vi "set_up_graph_control_properties.vi"(9 "Graph Properties":T2, 10 "viewing volume":dbl[](array[numeric]), 11 "3D Picture Control Reference":refnum<vi>) -> ()   [LabVIEW 2020, in "3DPC_SurfacePlot.xctl"]
uses:
  <vilib>/Native 3D Graph/xcontrol/3DPC_SurfacePlot.xctl
  <vilib>/Native 3D Graph/typedefs/prop_graph.ctl
  <vilib>/picture/3D Picture Control/NI_3D Picture Control.lvlib
panel:
  in  "View Direction":T1(ring)
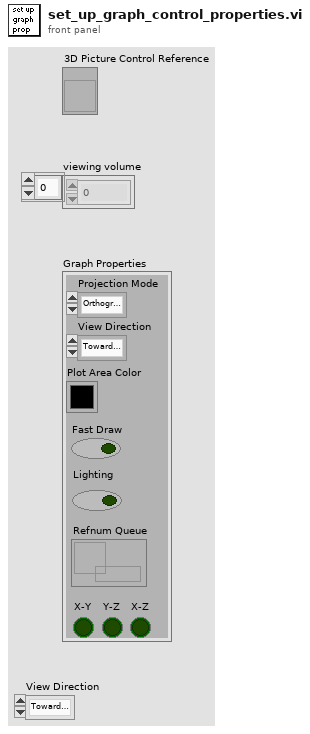
[diagram p1: front panel]
types:
  T1 = enum32{"Towards X-Y Plane", "Towards Y-Z Plane", "Towards X-Z Plane", "User Define"}
  T2 = typedef "3DPC_SurfacePlot.xctl/prop_graph.ctl" = cluster{"Projection Mode":enum16{"Orthographic", "Perspective"}, "View Direction":enum32{"Towards X-Y Plane", "Towards Y-Z Plane", "Towards X-Z Plane", "User Define"}, "Plot Area Color":u32, "Fast Draw":bool, "X-Y":bool, "Y-Z":bool, "X-Z":bool, "Lighting":bool, "Refnum Queue":refnum<queue>}
  T3 = enum16{"None", "Spherical", "Flying", "Oriented"}
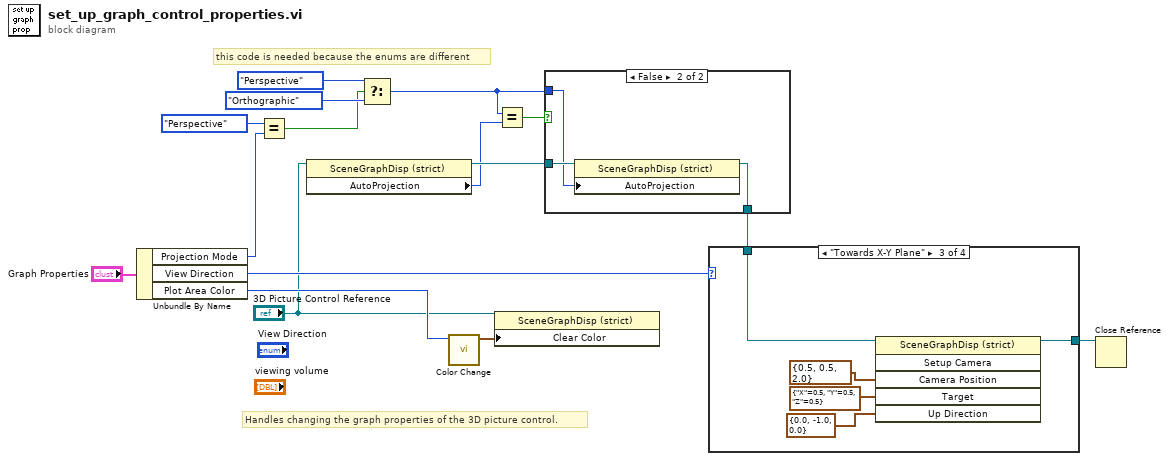
[diagram p0: block diagram]
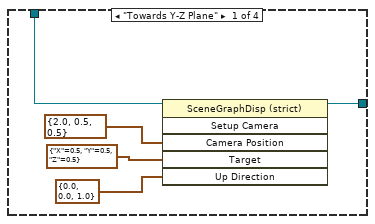
[diagram p2: hidden frame]
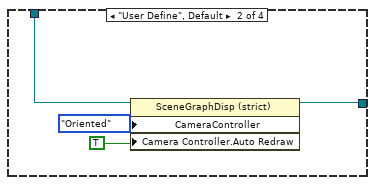
[diagram p3: hidden frame]
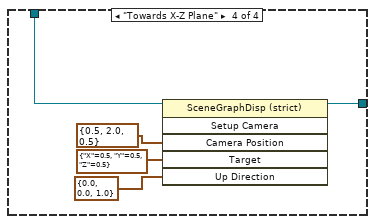
[diagram p4: hidden frame]
diagram:
  # "this code is needed because the enums are different"
  # "Handles changing the graph properties of the 3D picture control."
  n1 = Unbundle By Name("Graph Properties") -> ("Projection Mode"=w6:enum16{"Orthographic", "Perspective"}, "View Direction"=w15:T1, "Plot Area Color"=w14:u32)
  n2 = Equal?(x=enum16{"Orthographic", "Perspective"}."Perspective", y=w6) -> (x = y?=w4:bool)
  n3 = property class="SceneGraphDisp (strict)"(reference="3D Picture Control Reference") -> (reference out=w10:refnum<vi>, "AutoProjection"=w3:enum16{"None", "Perspective", "Orthographic"})  [unwired: 1 in, 1 out]
  n4 = Select(t=enum16{"None", "Perspective", "Orthographic"}."Perspective" ("Automatic Projection Mode"), s=w4, f=enum16{"None", "Perspective", "Orthographic"}."Orthographic" ("Automatic Projection Mode")) -> (s? t:f=w1:enum16{"None", "Perspective", "Orthographic"})
  n5 = call <vilib>:"Color Change.vi"("Color"=w14) -> ("RGBA"=w13:cluster{"R":sgl, "G":sgl, "B":sgl, "A":sgl})  [unwired: 1 in, 9 out]
  n6 = property on="Property Node" class="SceneGraphDisp (strict)"(reference="3D Picture Control Reference", "Clear Color"=w13) -> ()  [unwired: 1 in, 2 out]
  n7 = Equal?(x=w1, y=w3) -> (x = y?=w12:bool)
  n8 = case shown="False" w12 {
    tunnel: [w17 w18] -> w9
    tunnel: w10 -> [w17 w20]
    tunnel: w1 -> [_ w19]
    frame True {
    }
    frame False {
      n9 = property class="SceneGraphDisp (strict)"(reference=w20, "AutoProjection"=w19) -> (reference out=w18:refnum<vi>)  [unwired: 1 in, 1 out]
    }
  }
  n10 = case shown="\"Towards X-Y Plane\"" w15 {
    tunnel: [w22 w27 w30 w35] -> w2
    tunnel: w9 -> [w21 w28 w31 w36]
    frame "Towards Y-Z Plane" {
      n11 = invoke class="SceneGraphDisp (strict)" method="Setup Camera"(reference=w21, "Camera Position"=cluster{"X":sgl, "Y":sgl, "Z":sgl} {"X"=2.0, "Y"=0.5, "Z"=0.5}, "Target"=cluster{"X":sgl, "Y":sgl, "Z":sgl} {"X"=0.5, "Y"=0.5, "Z"=0.5} ("Camera Position"), "Up Direction"=cluster{"X":sgl, "Y":sgl, "Z":sgl} {"X"=0.0, "Y"=0.0, "Z"=1.0} ("Camera Position")) -> (reference out=w22:refnum<vi>)  [unwired: 2 in, 5 out]
    }
    frame "User Define", Default {
      n12 = property class="SceneGraphDisp (strict)"(reference=w28, "CameraController"=T3."Oriented" ("Camera Controller:Type"), "Camera Controller.Auto Redraw"=TRUE ("Camera Controller:Auto Redraw")) -> (reference out=w27:refnum<vi>)  [unwired: 1 in, 1 out]
    }
    frame "Towards X-Y Plane" {
      n13 = invoke class="SceneGraphDisp (strict)" method="Setup Camera"(reference=w31, "Camera Position"=cluster{"X":sgl, "Y":sgl, "Z":sgl} {"X"=0.5, "Y"=0.5, "Z"=2.0}, "Target"=cluster{"X":sgl, "Y":sgl, "Z":sgl} {"X"=0.5, "Y"=0.5, "Z"=0.5} ("Camera Position"), "Up Direction"=cluster{"X":sgl, "Y":sgl, "Z":sgl} {"X"=0.0, "Y"=-1.0, "Z"=0.0} ("Camera Position")) -> (reference out=w30:refnum<vi>)  [unwired: 2 in, 5 out]
    }
    frame "Towards X-Z Plane" {
      n14 = invoke class="SceneGraphDisp (strict)" method="Setup Camera"(reference=w36, "Camera Position"=cluster{"X":sgl, "Y":sgl, "Z":sgl} {"X"=0.5, "Y"=2.0, "Z"=0.5}, "Target"=cluster{"X":sgl, "Y":sgl, "Z":sgl} {"X"=0.5, "Y"=0.5, "Z"=0.5} ("Camera Position"), "Up Direction"=cluster{"X":sgl, "Y":sgl, "Z":sgl} {"X"=0.0, "Y"=0.0, "Z"=1.0} ("Camera Position")) -> (reference out=w35:refnum<vi>)  [unwired: 2 in, 5 out]
    }
  }
  n15 = Close Reference(reference=w2) -> ()  [unwired: 1 in, 1 out]
